vi "Set Burst Count.vi"(8 "error in (no error)":errorcluster, 10 "Burst Count":i32, 11 "VISA resource name":refnum<visa-resource-name>) -> (0 "error out":errorcluster, 3 "VISA resource name out":refnum<visa-resource-name>, 4 "Device Errors":cluster{"code":i32, "Text":string}[](array[cluster]))   [LabVIEW 2014, in "Stanford Research DG645 - Driver.lvlib"]
doc: "Burst Command: BURC i\nInstrument Error Check\n\nSet the burst count to i. When burst mode is enabled, the DG645 outputs burst count delay cycles per trigger."
uses:
  Stanford Research DG645 - Driver.lvlib
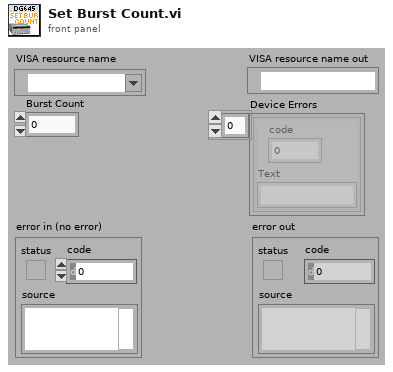
[diagram p1: front panel]
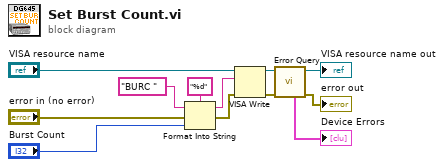
[diagram p0: block diagram]
diagram:
  n1 = Format Into String(format string="%d", initial string="BURC " ("command"), error in="error in (no error)", "Burst Count") -> (resulting string=w2:string, error out=w1:errorcluster)
  n2 = VISA Write(VISA resource name="VISA resource name", write buffer=w2, error in (no error)=w1) -> (VISA resource name out=w8:refnum<visa-resource-name>, error out=w5:errorcluster)  [unwired: 1 out]
  n3 = call "Error Query.vi"("error in (no error)"=w5, "VISA resource name"=w8) -> ("error out"=→"error out":errorcluster, "VISA resource name out"=→"VISA resource name out":refnum<visa-resource-name>, "Device Errors"=→"Device Errors":cluster{"code":i32, "Text":string}[])  [unwired: 7 in]
